vi "Teleop.vi"(10 "Match Info":T1={"Autonomous Elapsed Seconds"=0.0, "TeleOp Elapsed Seconds"=0.0, "Disabled Elapsed Seconds"=0.0, "Visited Autonomous"=FALSE, "Visited TeleOp"=FALSE, "Visited Disabled"=FALSE, "Autonomous Settings"={"Autonomous Style"=enum."Independent", "VI Refnum"=refnum}}, 11 "Call Context":T2) -> ()   [LabVIEW 2014]
doc: "This VI is called for each TeleOp packet received from the DS where the robot is not disabled. It is often used to read from the joysticks and update I/O or to update setpoints for timed control loops. It should complete and return within 20 milliseconds or it may miss DS packets."
uses:
  <vilib>/Rock Robotics/Network Tables/SD Write Numeric Array.vi
  <vilib>/Rock Robotics/WPI/RobotDrive/WPI_RobotDriveArcadeDrive_Standard(NoSaturation).vi
  <vilib>/Rock Robotics/WPI/Solenoid/WPI_SolenoidSetEnum.vi
  <vilib>/Rock Robotics/WPI/Solenoid/WPI_SolenoidValue.ctl
  <vilib>/Rock Robotics/WPI/DriverStation/WPI_DriverStationMatch Info.ctl
  <vilib>/Rock Robotics/WPI/DriverStation/WPI_DriverStationDerivedRobotMode.ctl
panel:
  out "LS 4":bool
  out "Front Lift Raw Output 2":dbl
  out "LS 3":bool
  out "LS 2":bool
  out "LS 1":bool
  out "Axes[5]":dbl
  out "Axes[1]":dbl
  out "Front Lift Raw Output":dbl
  out "Intake Wheel Raw Output":dbl
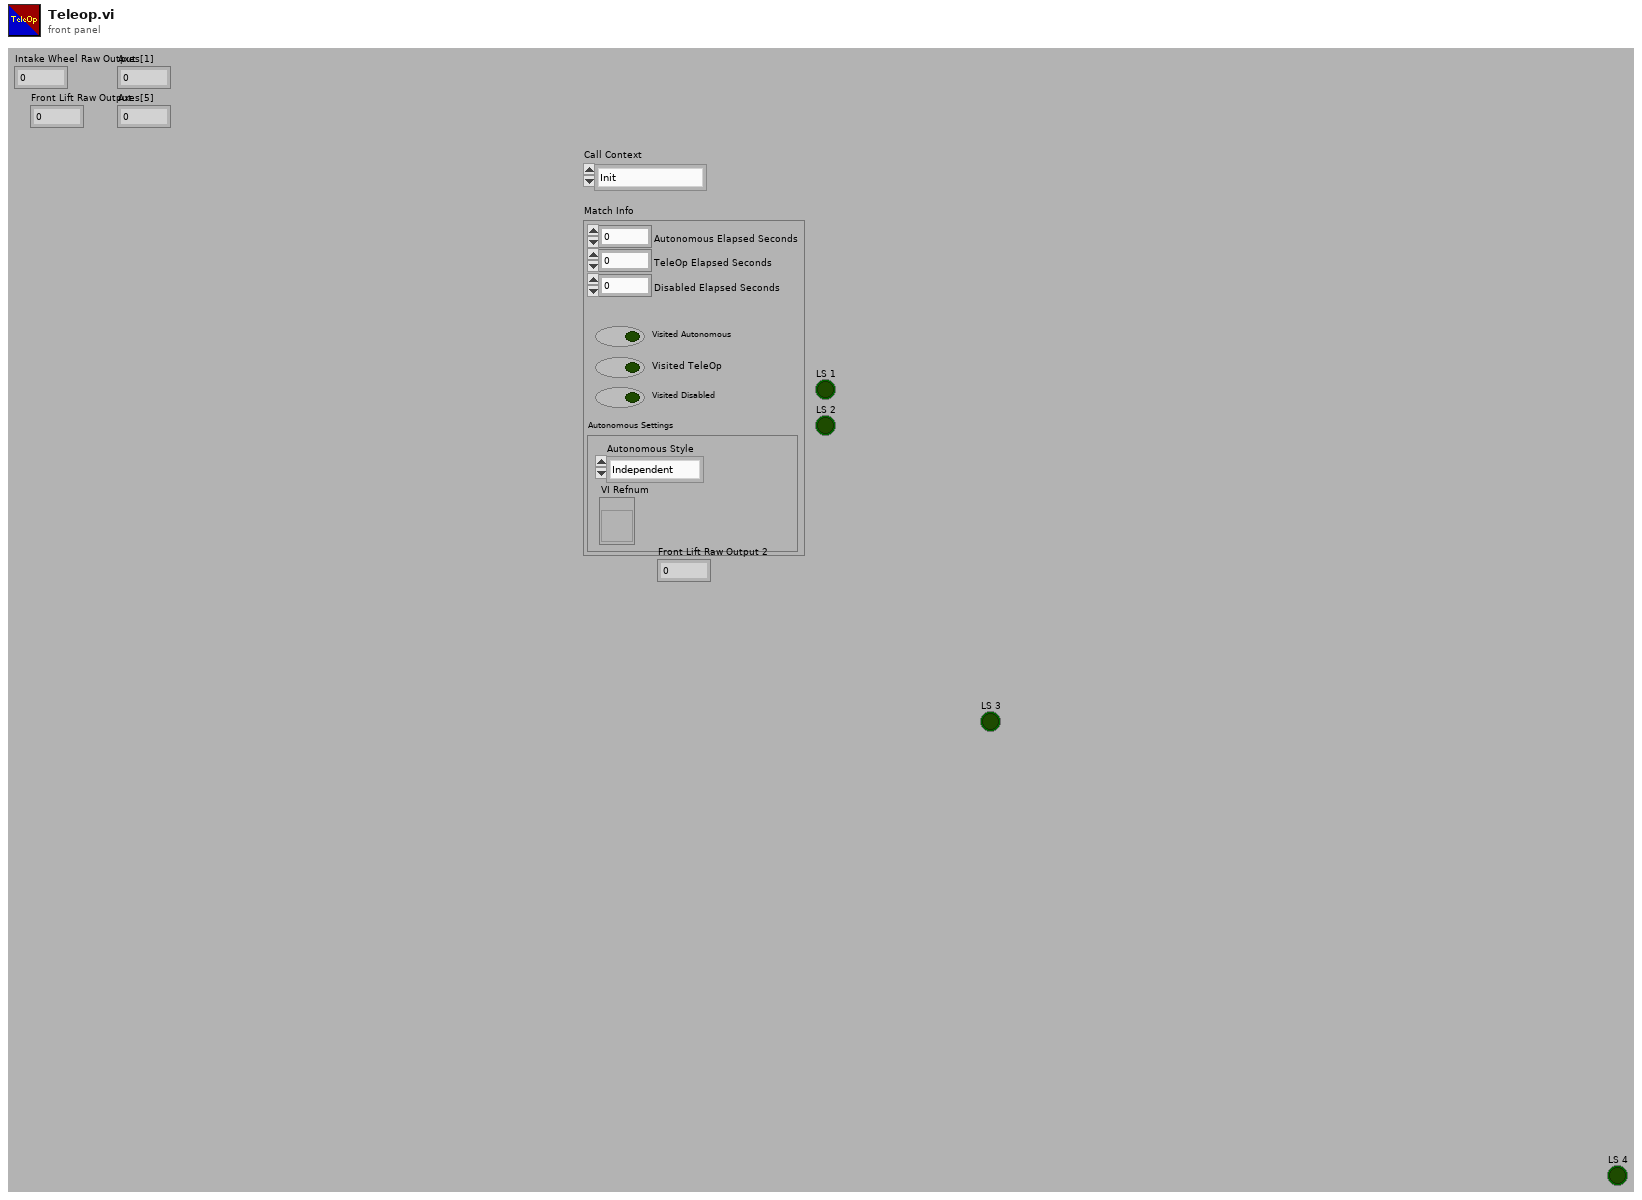
[diagram p1: front panel]
types:
  T1 = typedef "WPI_DriverStationMatch Info.ctl" = cluster{"Autonomous Elapsed Seconds":dbl, "TeleOp Elapsed Seconds":dbl, "Disabled Elapsed Seconds":dbl, "Visited Autonomous":bool, "Visited TeleOp":bool, "Visited Disabled":bool, "Autonomous Settings":cluster{"Autonomous Style":enum16{"Iterative", "Independent"}, "VI Refnum":refnum<vi>}}
  T2 = typedef "WPI_DriverStationDerivedRobotMode.ctl" = enum16{"Init", "Execute", "Stop"}
  T3 = typedef "WPI_SolenoidValue.ctl" = enum16{"Off", "On", "Forward", "Reverse"}
  T4 = typedef "WPI_JoystickDevRef.ctl" = cluster{"Device":T5}
  T5 = typedef "WPI_JoystickDeviceEnum.ctl" = enum16{"USB 0", "USB 1", "USB 2", "USB 3", "USB 4", "USB 5"}
  T6 = cluster{"Axes[0]":dbl, "Axes[1]":dbl, "Axes[2]":dbl, "Axes[3]":dbl, "Axes[4]":dbl, "Axes[5]":dbl, "Axes[6]":dbl, "Axes[7]":dbl, "Axes[8]":dbl}
  T7 = cluster{"Buttons[0]":bool, "Buttons[1]":bool, "Buttons[2]":bool, "Buttons[3]":bool, "Buttons[4]":bool, "Buttons[5]":bool, "Buttons[6]":bool, "Buttons[7]":bool, "Buttons[8]":bool}
  T8 = typedef "WPI_RobotDriveDevRef.ctl" = cluster{"DevStatus":errorcluster, "Motors[]":T9[], "Square Inputs":bool, "Max Output":dbl}
  T9 = typedef "WPI_MotorControlDeviceRef.ctl" = cluster{"DeviceStatus":errorcluster, "Type":T10, "PWM":cluster{"Controller":T11, "PWM Channel":T12, "DeadBand":T13}, "CAN":cluster{"Device Number":u8, "Control Mode":T14, "Semaphore":T15, "Max Vout":dbl, "TalonSRX Control Mode":T16}, "Invert":bool, "TransformRef":T17, "InvTransformRef":T17}
  T10 = typedef "WPI_MotorControlType.ctl" = enum16{"PWM", "CAN", "CANTalonSRX"}
  T11 = typedef "FPGA_TypedefDigitalModule.ctl" = enum16{"Controller 1"}
  T12 = typedef "FPGA_DIOPWMChannel.ctl" = enum8{"PWM 0", "PWM 1", "PWM 2", "PWM 3", "PWM 4", "PWM 5", "PWM 6", "PWM 7", "PWM 8", "PWM 9", "PWM MXP 0", "PWM MXP 1", "PWM MXP 2", "PWM MXP 3", "PWM MXP 4", "PWM MXP 5", "PWM MXP 6", "PWM MXP 7", "PWM MXP 8", "PWM MXP 9", "Invalid"}
  T13 = typedef "WPI_PWMDeadband.ctl" = cluster{"Name":string, "maxPositivePwm":i32, "minPositivePwm":i32, "centerPwm":i32, "maxNegativePwm":i32, "minNegativePwm":i32, "angularRange":u16}
  T14 = typedef "WPI_CANJaguar_ControlMode.ctl" = enum8{"Percent VBus", "Current", "Speed", "Position", "Voltage"}
  T15 = typedef "Semaphore RefNum" = refnum<k1>
  T16 = typedef "WPI_CANTalonSRX_APIControlMode.ctl" = enum8{"Percent VBus", "Speed", "Position", "Slave", "Unchanged / Invalid"}
  T17 = typedef "WPI_PWMTransform_ConPane.ctl" = refnum<vi>
  T18 = typedef "WPI_SwitchDevRef.ctl" = cluster{"DevStatus":errorcluster, "DIO Channel":T19, "Controller":T11, "CntIndex":T20, "Normally Closed":bool}
  T19 = typedef "FPGA_DIOChannel.ctl" = enum8{"DIO 0", "DIO 1", "DIO 2", "DIO 3", "DIO 4", "DIO 5", "DIO 6", "DIO 7", "DIO 8", "DIO 9", "DIO MXP 0", "DIO MXP 1", "DIO MXP 2", "DIO MXP 3", "DIO MXP 4", "DIO MXP 5", "DIO MXP 6", "DIO MXP 7", "DIO MXP 8", "DIO MXP 9", "DIO MXP 10", "DIO MXP 11", "DIO MXP 12", "DIO MXP 13", "DIO MXP 14", "DIO MXP 15", "Invalid"}
  T20 = typedef "FPGA_CounterCtrSystemIndex.ctl" = enum8{"Ctr 0", "Ctr 1", "Ctr 2", "Ctr 3", "Ctr 4", "Ctr 5", "Ctr 6", "Ctr 7", "Invalid"}
  T21 = typedef "WPI_SolenoidDevRef.ctl" = cluster{"DevStatus":errorcluster, "Pneumatics Control Module":u8, "Forward Solenoid Channel":T22, "Reverse Solenoid Channel":T22}
  T22 = typedef "WPI_SolenoidChannel.ctl" = enum8{"Solenoid 0", "Solenoid 1", "Solenoid 2", "Solenoid 3", "Solenoid 4", "Solenoid 5", "Solenoid 6", "Solenoid 7", "Invalid"}
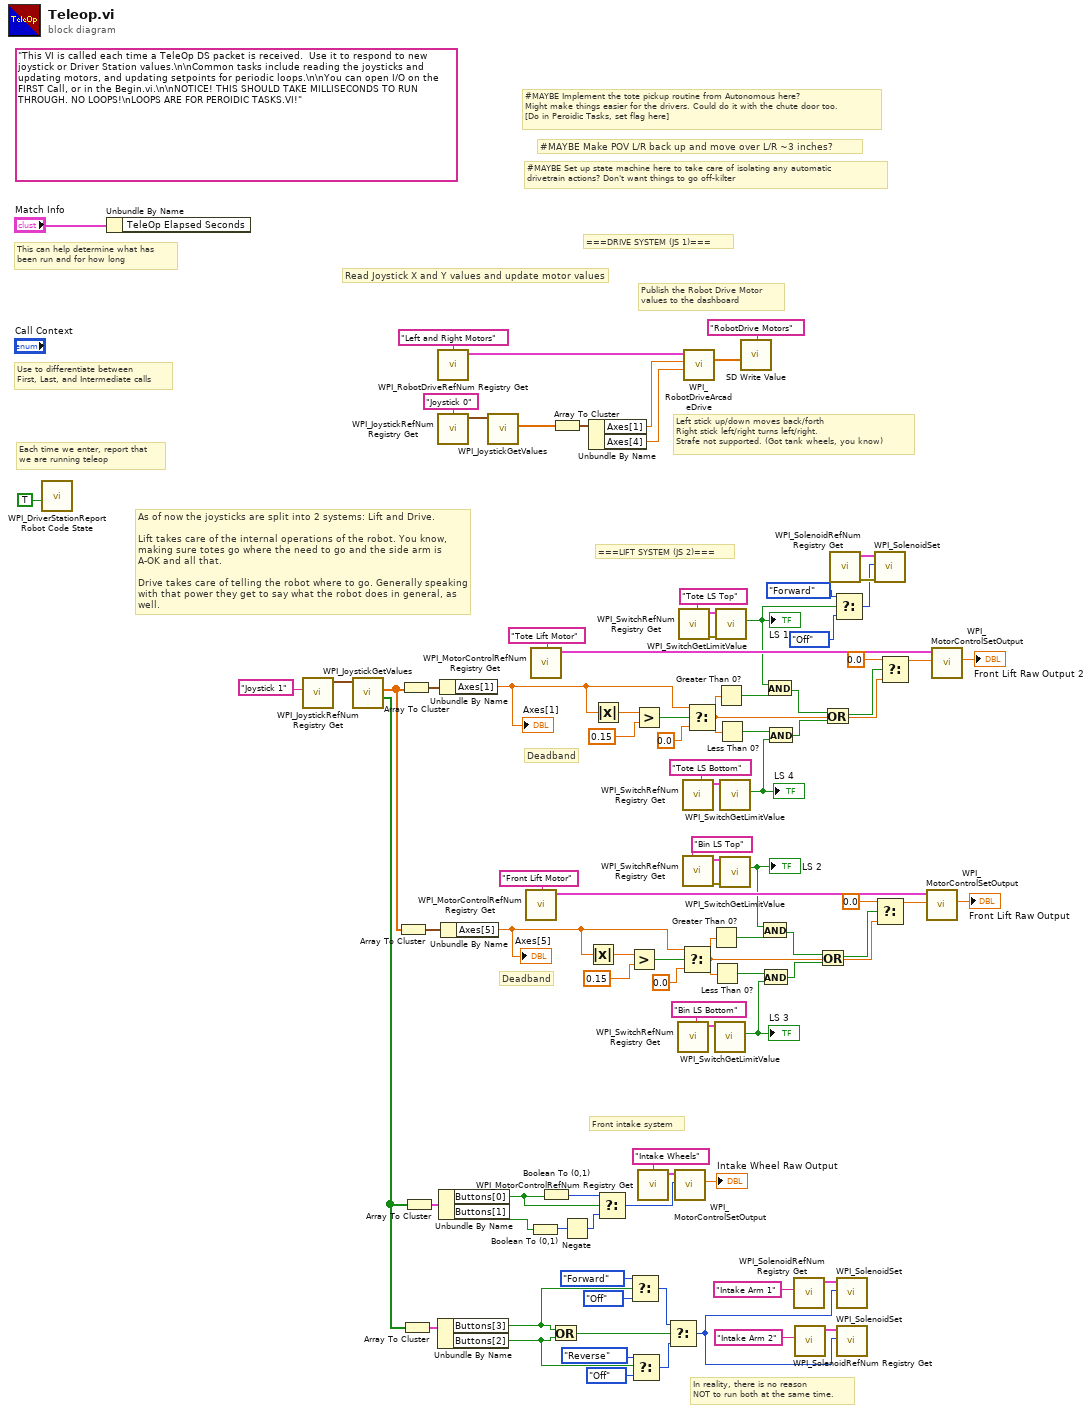
[diagram p0: block diagram]
diagram:
  (unwired) "This VI is called each time a TeleOp DS packet is received.  Use it to respond to new joystick or Driver Station values.\n\nCommon tasks include reading the joysticks and updating motors, and updating setpoints for periodic loops.\n\nYou can open I/O on the FIRST Call, or in the Begin.vi.\n\nNOTICE! THIS SHOULD TAKE MILLISECONDS TO RUN THROUGH. NO LOOPS!\nLOOPS ARE FOR PEROIDIC TASKS.VI!"
  # "Deadband"
  # "#MAYBE Set up state machine here to take care of isolating any automatic\ndrivetrain actions? Don't want things to go off-kilter"
  # "Front intake system"
  # "As of now the joysticks are split into 2 systems: Lift and Drive.\n\nLift takes care of the internal operations of the robot. You know,\nmaking sure totes go where the need to go and the side arm is\nA-OK and all that.\n\nDrive takes care of telling the robot where to go. Generally speaking\nwith that power they get to say what the robot does in general, as well."
  # "===LIFT SYSTEM (JS 2)==="
  # "===DRIVE SYSTEM (JS 1)==="
  # "In reality, there is no reason \nNOT to run both at the same time."
  # "#MAYBE Make POV L/R back up and move over L/R ~3 inches?"
  # "Left stick up/down moves back/forth\nRight stick left/right turns left/right.\nStrafe not supported. (Got tank wheels, you know)"
  # "#MAYBE Implement the tote pickup routine from Autonomous here?\nMight make things easier for the drivers. Could do it with the chute door too.\n[Do in Peroidic Tasks, set flag here]"
  # "Deadband"
  # "Publish the Robot Drive Motor\nvalues to the dashboard"
  # "Each time we enter, report that\nwe are running teleop"
  # "Use to differentiate between\nFirst, Last, and Intermediate calls"
  # "This can help determine what has\nbeen run and for how long"
  # "Read Joystick X and Y values and update motor values"
  n1 = call <vilib>:"WPI_DriverStationReport Robot Code State.vi"("TeleOp"=TRUE ("Autonomous")) -> ()  [unwired: 10 in, 1 out]
  n2 = Unbundle By Name("Match Info") -> ()  [unwired: 1 out]
  n3 = call <vilib>:"WPI_JoystickRefNum Registry Get.vi"("refnum name"="Joystick 1") -> ("JoystickDevRef"=w81:T4)  [unwired: 1 in, 9 out]
  n4 = call <vilib>:"WPI_JoystickGetValues.vi"("JoystickDevRef"=w81) -> ("Buttons"=w43:bool[], "Axes"=w40:dbl[])  [unwired: 6 in, 3 out]
  n5 = Array To Cluster(array=w40) -> (cluster=w39:T6)
  n6 = Array To Cluster(array=w40) -> (cluster=w80:T6)
  n7 = Array To Cluster(array=w43) -> (cluster=w79:T7)
  n8 = Array To Cluster(array=w43) -> (cluster=w65:T7)
  n9 = call <vilib>:"WPI_RobotDriveRefNum Registry Get.vi"("refnum name"="Left and Right Motors") -> ("RobotDriveDevRef"=w92:T8)  [unwired: 1 in, 9 out]
  n10 = call <vilib>:"WPI_JoystickRefNum Registry Get.vi"("refnum name"="Joystick 0") -> ("JoystickDevRef"=w90:T4)  [unwired: 1 in, 9 out]
  n11 = Unbundle By Name(w79) -> ("Buttons[3]"=w37:bool, "Buttons[2]"=w36:bool)
  n12 = Unbundle By Name(w65) -> ("Buttons[0]"=w68:bool, "Buttons[1]"=w66:bool)
  n13 = Unbundle By Name(w80) -> ("Axes[1]"=w8:dbl)
  "Axes[1]" <- w8
  n14 = Unbundle By Name(w39) -> ("Axes[5]"=w38:dbl)
  "Axes[5]" <- w38
  n15 = call <vilib>:"WPI_JoystickGetValues.vi"("JoystickDevRef"=w90) -> ("Axes"=w86:dbl[])  [unwired: 6 in, 4 out]
  n16 = call <vilib>:"WPI_MotorControlRefNum Registry Get.vi"("refnum name"="Front Lift Motor") -> ("MotorControlDevRef"=w64:T9)  [unwired: 9 in, 1 out]
  n17 = Boolean To (0,1)(Boolean=w66) -> (0, 1=w42:i16)
  n18 = call <vilib>:"WPI_MotorControlRefNum Registry Get.vi"("refnum name"="Tote Lift Motor") -> ("MotorControlDevRef"=w25:T9)  [unwired: 9 in, 1 out]
  n19 = Boolean To (0,1)(Boolean=w68) -> (0, 1=w67:i16)
  n20 = Or(x=w37, y=w36) -> (x .or. y?=w35:bool)
  n21 = Array To Cluster(array=w86) -> (cluster=w85:T6)
  n22 = Negate(x=w42) -> (-x=w41:i16)
  n23 = Absolute Value(x=w38) -> (abs(x)=w57:dbl)
  n24 = Unbundle By Name(w85) -> ("Axes[1]"=w84:dbl, "Axes[4]"=w83:dbl)
  n25 = Absolute Value(x=w8) -> (abs(x)=w23:dbl)
  n26 = Select(t=w67, s=w68, f=w41) -> (s? t:f=w60:i16)
  n27 = Greater?(x=w57, y=0.15) -> (0:w55:bool)
  n28 = Select(t=WPI_SolenoidValue."Forward" ("Value"), s=w37, f=WPI_SolenoidValue."Off") -> (s? t:f=w69:T3)
  n29 = Select(t=WPI_SolenoidValue."Reverse" ("f"), s=w36, f=WPI_SolenoidValue."Off") -> (s? t:f=w70:T3)
  n30 = Greater?(x=w23, y=0.15) -> (0:w21:bool)
  n31 = call <vilib>:"WPI_MotorControlRefNum Registry Get.vi"("refnum name"="Intake Wheels") -> ("MotorControlDevRef"=w62:T9)  [unwired: 9 in, 1 out]
  n32 = Select(t=w69, s=w35, f=w70) -> (s? t:f=w50:T3)
  n33 = call <vilib>:"WPI_MotorControlSetOutput.vi"("Output"=w60, "MotorControlDevRef"=w62) -> ("Motor Output"=→"Intake Wheel Raw Output":dbl)  [unwired: 7 in, 2 out]
  n34 = call <vilib>:"WPI_SwitchRefNum Registry Get.vi"("refnum name"="Bin LS Bottom") -> ("SwitchDevRef"=w33:T18)  [unwired: 9 in, 1 out]
  n35 = call <vilib>:"WPI_SwitchRefNum Registry Get.vi"("refnum name"="Tote LS Top") -> ("error out"=w52:errorcluster, "SwitchDevRef"=w51:T18)  [unwired: 9 in]
  n36 = Select(t=w38, s=w55, f=0.0 ("t")) -> (s? t:f=w26:dbl)
  n37 = call <vilib>:"WPI_SwitchRefNum Registry Get.vi"("refnum name"="Tote LS Bottom") -> ("SwitchDevRef"=w16:T18)  [unwired: 9 in, 1 out]
  n38 = call <vilib>:"WPI_SwitchRefNum Registry Get.vi"("refnum name"="Bin LS Top") -> ("error out"=w48:errorcluster, "SwitchDevRef"=w47:T18)  [unwired: 9 in]
  n39 = call-poly <vilib>:"WPI_RobotDriveArcadeDrive.vi"("Y axis value"=w83, "X axis value"=w84, "RobotDriveDevRef"=w92) -> ("Motor Values"=w87:dbl[])  [unwired: 6 in, 2 out]
  n40 = Select(t=w8, s=w21, f=0.0 ("t")) -> (s? t:f=w9:dbl)
  n41 = Greater Than 0?(x=w26) -> (x > 0?=w45:bool)
  n42 = Less Than 0?(x=w26) -> (x < 0?=w31:bool)
  n43 = call <vilib>:"WPI_SwitchGetLimitValue.vi"("SwitchDevRef"=w33) -> ("Switch Pressed"=w32:bool)  [unwired: 8 in, 2 out]
  "LS 3" <- w32
  n44 = call <vilib>:"WPI_SwitchGetLimitValue.vi"("error in (no error)"=w52, "SwitchDevRef"=w51) -> ("Switch Pressed"=w4:bool)  [unwired: 7 in, 2 out]
  "LS 1" <- w4
  n45 = Greater Than 0?(x=w9) -> (x > 0?=w19:bool)
  n46 = Less Than 0?(x=w9) -> (x < 0?=w14:bool)
  n47 = call <vilib>:"WPI_SwitchGetLimitValue.vi"("SwitchDevRef"=w16) -> ("Switch Pressed"=w15:bool)  [unwired: 8 in, 2 out]
  "LS 4" <- w15
  n48 = call <vilib>:"WPI_SwitchGetLimitValue.vi"("error in (no error)"=w48, "SwitchDevRef"=w47) -> ("Switch Pressed"=w46:bool)  [unwired: 7 in, 2 out]
  "LS 2" <- w46
  n49 = call-poly <vilib>:"SD Write Value.vi"("Numeric Array"=w87, "Name"="RobotDrive Motors") -> ()  [unwired: 8 in, 2 out]
  n50 = And(x=w46, y=w45) -> (x .and. y?=w30:bool)
  n51 = And(x=w31, y=w32) -> (x .and. y?=w29:bool)
  n52 = And(x=w4, y=w19) -> (x .and. y?=w13:bool)
  n53 = And(x=w14, y=w15) -> (x .and. y?=w12:bool)
  n54 = call <vilib>:"WPI_SolenoidRefNum Registry Get.vi"("refnum name"="Intake Arm 1") -> ("SolenoidDevRef"=w77:T21)  [unwired: 9 in, 1 out]
  n55 = call <vilib>:"WPI_SolenoidRefNum Registry Get.vi"("refnum name"="Intake Arm 2") -> ("SolenoidDevRef"=w75:T21)  [unwired: 9 in, 1 out]
  n56 = Or(x=w30, y=w29) -> (x .or. y?=w28:bool)
  n57 = Or(x=w13, y=w12) -> (x .or. y?=w11:bool)
  n58 = call <vilib>:"WPI_SolenoidRefNum Registry Get.vi"() -> ("error out"=w6:errorcluster, "SolenoidDevRef"=w5:T21)  [unwired: 10 in]
  n59 = Select(t=WPI_SolenoidValue."Forward" ("Value"), s=w4, f=WPI_SolenoidValue."Off" ("Value")) -> (s? t:f=w1:T3)
  n60 = call-poly <vilib>:"WPI_SolenoidSet.vi"("Value"=w50, "SolenoidDevRef"=w77) -> ()  [unwired: 8 in, 2 out]
  n61 = call-poly <vilib>:"WPI_SolenoidSet.vi"("Value"=w50, "SolenoidDevRef"=w75) -> ()  [unwired: 8 in, 2 out]
  n62 = call-poly <vilib>:"WPI_SolenoidSet.vi"("error in (no error)"=w6, "Value"=w1, "SolenoidDevRef"=w5) -> ()  [unwired: 7 in, 2 out]
  n63 = Select(t=0.0, s=w28, f=w26) -> (s? t:f=w27:dbl)
  n64 = Select(t=0.0, s=w11, f=w9) -> (s? t:f=w10:dbl)
  n65 = call <vilib>:"WPI_MotorControlSetOutput.vi"("Output"=w27, "MotorControlDevRef"=w64) -> ("Motor Output"=→"Front Lift Raw Output":dbl)  [unwired: 7 in, 2 out]
  n66 = call <vilib>:"WPI_MotorControlSetOutput.vi"("Output"=w10, "MotorControlDevRef"=w25) -> ("Motor Output"=→"Front Lift Raw Output 2":dbl)  [unwired: 7 in, 2 out]
